vi "MicroPulse - dof decoder.vi"(0 "dof":u32) -> (2 "String":string, 3 "DOF":T1=enum."8-bit Mode" caption="dof")   [LabVIEW 2026, in "MicroPulse_Driver.lvlib"]
uses:
  MicroPulse_Driver.lvlib
  Public/Data/Datatypes/MP - data output format.ctl
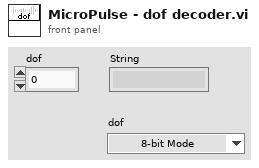
[diagram p1: front panel]
types:
  T1 = typedef "MicroPulse_Driver.lvlib/MP - data output format.ctl" = enum16{"", "8-bit Mode", "10-bit Mode", "12-bit Mode", "16-bit Mode", "8-bit Log Mode", "12-bit Packed Mode"}
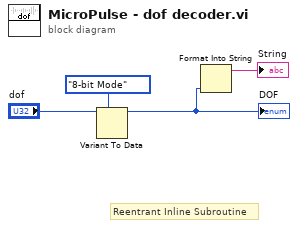
[diagram p0: block diagram]
diagram:
  # "Reentrant Inline Subroutine"
  n1 = Variant To Data(type=MP_-_data_output_format."8-bit Mode" ("DOF"), Variant="dof") -> (data=w1:T1)  [unwired: 1 in, 1 out]
  "DOF" <- w1
  n2 = Format Into String(w1) -> (resulting string=→"String":string)  [unwired: 3 in, 1 out]
